vi "Periodic Tasks.vi"(8 "error in (no error)":errorcluster) -> ()   [LabVIEW 2011]
doc: "This VI runs in parallel to other tasks. It can contain as many user-defined periodic loops as you need. These can carry out PID or other sorts of timed response."
uses:
  <vilib>/Rock Robotics/SystemInterfaces/Utilities/FPGA_UtilitiesLED State.ctl
  <vilib>/Rock Robotics/SystemInterfaces/Utilities/FPGA_UtilitiesLED Source.ctl
  Robot Global Data.vi
panel:
  out "Autonomous Switch":dbl
  out "Encoder Direction 4":string="Backward"
  out "Encoder Alarm Status 4":string="Encoder Moving"
  in  "stop 4":bool
  out "Encoder Distance 4":dbl
  out "Encoder Rate (distance/sec) 4":dbl
  out "Encoder Direction 3":string="Backward"
  out "Encoder Alarm Status 3":string="Encoder Moving"
  in  "Reset Encoder? 3":bool
  in  "stop 3":bool
  out "Encoder Distance 3":dbl
  out "Encoder Rate (distance/sec) 3":dbl
  out "Encoder Direction 2":string="Forward"
  out "Encoder Alarm Status 2":string="Encoder Stopped"
  in  "Reset Encoder? 2":bool
  in  "stop 2":bool
  out "Encoder Distance 2":dbl=1.0
  out "Encoder Rate (distance/sec) 2":dbl
  out "Encoder Direction":string="Forward"
  out "Encoder Alarm Status":string="Encoder Stopped"
  in  "Reset Encoder?":bool
  in  "stop":bool
  out "Encoder Distance":dbl=1.0
  out "Encoder Rate (distance/sec)":dbl
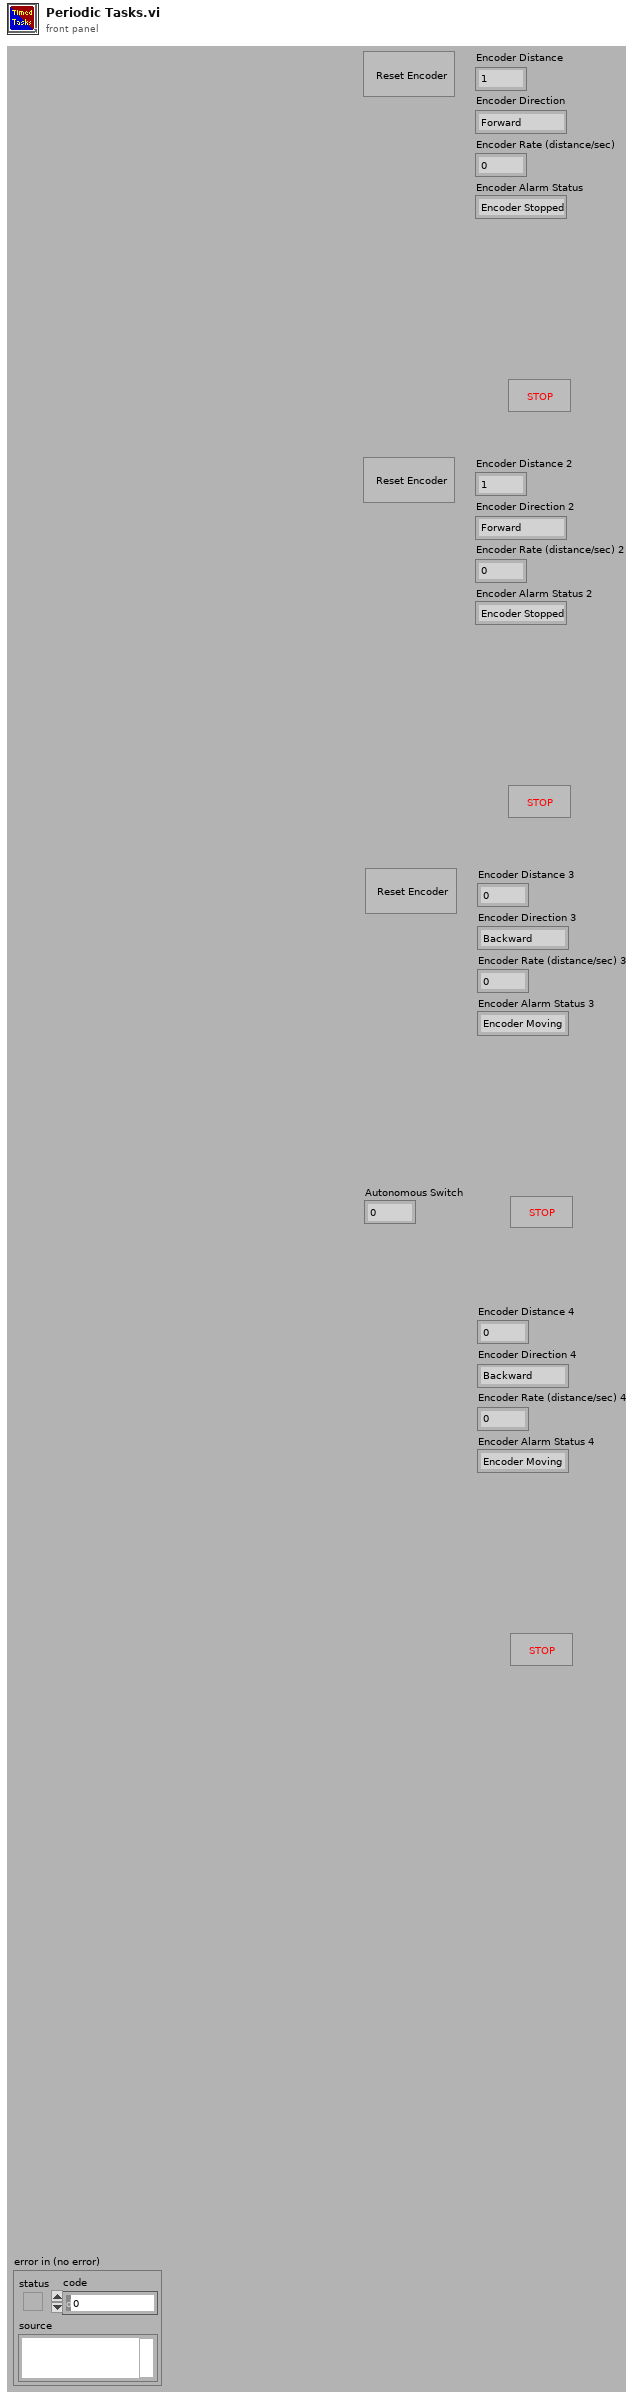
[diagram p1: front panel]
types:
  T1 = typedef "FPGA_UtilitiesLED State.ctl" = enum16{"Off", "On", "Toggle"}
  T2 = typedef "FPGA_UtilitiesLED Source.ctl" = enum16{"User LED", "FPGA LED"}
  T3 = enum16{"Shoot", "Load", "Arm", "Nothing", "Reverse", "ShootAll"}
  T4 = typedef "WPI_DigitalInputDevRef.ctl" = cluster{"DevStatus":errorcluster, "DIO Channel":T5, "Digital Module":T6}
  T5 = typedef "FPGA_DIOChannel.ctl" = enum8{"DIO 1", "DIO 2", "DIO 3", "DIO 4", "DIO 5", "DIO 6", "DIO 7", "DIO 8", "DIO 9", "DIO 10", "DIO 11", "DIO 12", "DIO 13", "DIO 14", "Invalid"}
  T6 = typedef "FPGA_TypedefDigitalModule.ctl" = enum16{"Digital Module 1", "Digital Module 2"}
  T7 = typedef "WPI_EncoderDevRef.ctl" = cluster{"DevStatus":errorcluster, "EncoderIndex":T8, "CounterIndex":T9, "DistancePerCount":dbl, "Decoding Type":T10}
  T8 = typedef "FPGA_EncoderIdx.ctl" = enum8{"Enc 0", "Enc 1", "Enc 2", "Enc 3", "Invalid"}
  T9 = typedef "FPGA_CounterCtrSystemIndex.ctl" = enum8{"Ctr 0", "Ctr 1", "Ctr 2", "Ctr 3", "Ctr 4", "Ctr 5", "Ctr 6", "Ctr 7", "Invalid"}
  T10 = typedef "WPI_EncoderType.ctl" = enum16{"1x", "2x", "4x"}
  T11 = typedef "WPI_MotorControlDeviceRef.ctl" = cluster{"DeviceStatus":errorcluster, "Type":enum16{"PWM", "CAN"}, "PWM":cluster{"Digital Module":T6, "PWM Channel":T12, "DeadBand":T13}, "CAN":cluster{"Device Number":u8, "Control Mode":T14, "Semaphore":T15, "Max Vout":dbl}, "Invert":bool, "TransformRef":T16, "InvTransformRef":T16}
  T12 = typedef "FPGA_DIOPWMChannel.ctl" = enum8{"PWM 1", "PWM 2", "PWM 3", "PWM 4", "PWM 5", "PWM 6", "PWM 7", "PWM 8", "PWM 9", "PWM 10", "Invalid"}
  T13 = typedef "WPI_PWMDeadband.ctl" = cluster{"Name":string, "maxPositivePwm":i32, "minPositivePwm":i32, "centerPwm":i32, "maxNegativePwm":i32, "minNegativePwm":i32, "angularRange":u16}
  T14 = typedef "WPI_CANJaguar_ControlMode.ctl" = enum8{"Percent VBus", "Current", "Speed", "Position", "Voltage"}
  T15 = typedef "Semaphore RefNum" = refnum<k1>
  T16 = typedef "WPI_PWMTransform_ConPane.ctl" = refnum<vi>
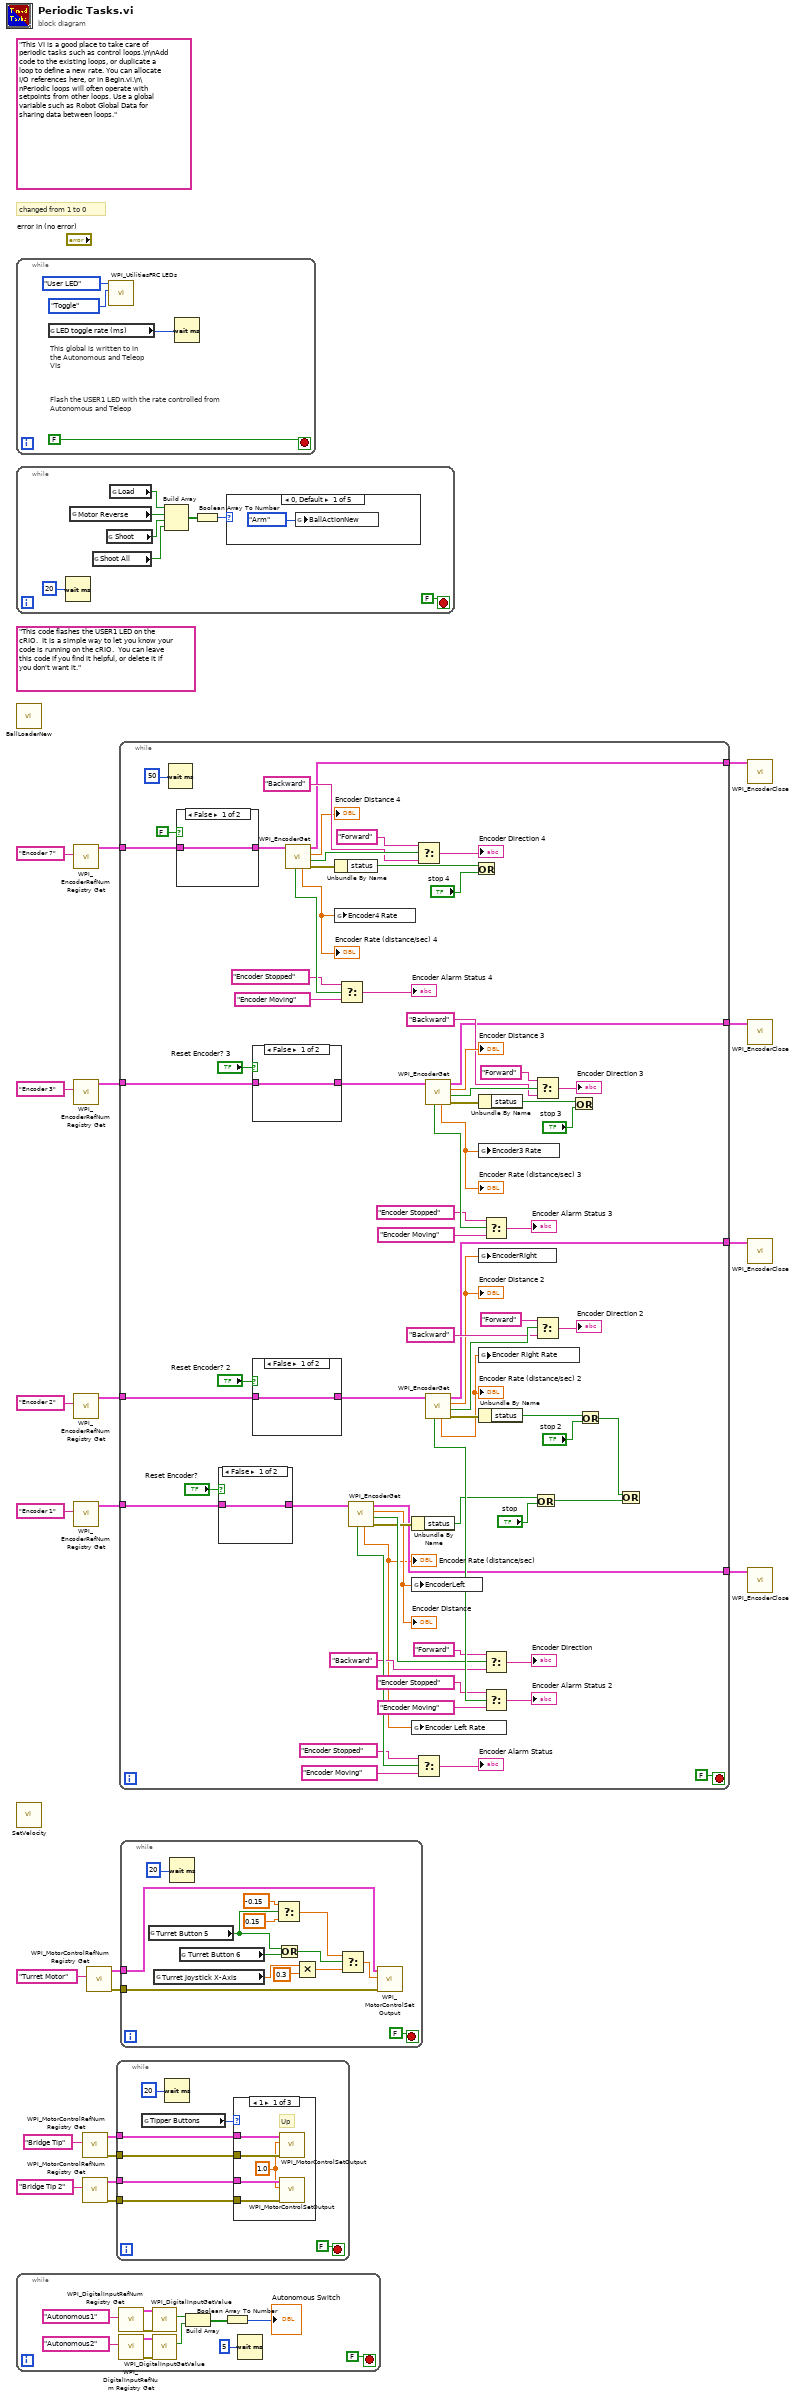
[diagram p0: block diagram]
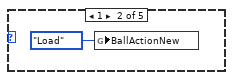
[diagram p2: hidden frame]
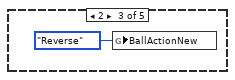
[diagram p3: hidden frame]
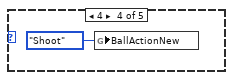
[diagram p4: hidden frame]
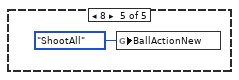
[diagram p5: hidden frame]
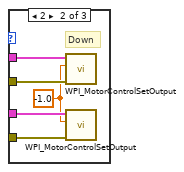
[diagram p6: hidden frame]
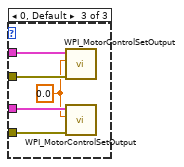
[diagram p7: hidden frame]
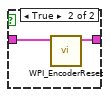
[diagram p8: hidden frame]
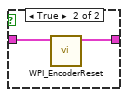
[diagram p9: hidden frame]
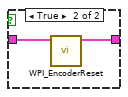
[diagram p10: hidden frame]
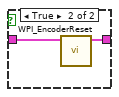
[diagram p11: hidden frame]
diagram:
  (unwired) "This VI is a good place to take care of periodic tasks such as control loops.\n\nAdd code to the existing loops, or duplicate a loop to define a new rate. You can allocate I/O references here, or in Begin.vi.\n\nPeriodic loops will often operate with setpoints from other loops. Use a global variable such as Robot Global Data for sharing data between loops."
  (unwired) "This code flashes the USER1 LED on the cRIO.  It is a simple way to let you know your code is running on the cRIO.  You can leave this code if you find it helpful, or delete it if you don't want it."
  # "changed from 1 to 0"
  n1 = while {
    stop <- FALSE stop-if-true
    # "This global is written to in the Autonomous and Teleop VIs"
    # "Flash the USER1 LED with the rate controlled from Autonomous and Teleop"
    n2 = global read "Robot Global Data.vi" "LED toggle rate (ms)"() -> (w22:u32)
    n3 = call <vilib>:"WPI_UtilitiesFRC LEDs.vi"("State"=FPGA_UtilitiesLED_State."Toggle", "LED Type"=FPGA_UtilitiesLED_Source."User LED") -> ()  [unwired: 1 in, 9 out]
    n4 = Wait (ms)(milliseconds to wait=w22) -> ()  [unwired: 1 out]
  }
  n5 = while {
    stop <- FALSE stop-if-true
    n6 = Wait (ms)(milliseconds to wait=u32 20) -> ()  [unwired: 1 out]
    n7 = global read "Robot Global Data.vi" "Motor Reverse"() -> (w31:bool)
    n8 = global read "Robot Global Data.vi" "Shoot All"() -> (w29:bool)
    n9 = global read "Robot Global Data.vi" "Shoot"() -> (w30:bool)
    n10 = global read "Robot Global Data.vi" "Load"() -> (w32:bool)
    n11 = Build Array(w32, w31, w30, w29) -> (w33:bool[])
    n12 = Boolean Array To Number(Boolean array=w33) -> (number=w28:u32)
    n13 = case shown="0, Default" w28 {
      frame 0, Default {
        n14 = global write "Robot Global Data.vi" "BallActionNew"(T3."Arm" ("BallActionNew")) -> ()
      }
      frame 1 {
        n15 = global write "Robot Global Data.vi" "BallActionNew"(T3."Load" ("BallActionNew")) -> ()
      }
      frame 2 {
        n16 = global write "Robot Global Data.vi" "BallActionNew"(T3."Reverse" ("BallActionNew")) -> ()
      }
      frame 4 {
        n17 = global write "Robot Global Data.vi" "BallActionNew"(T3."Shoot" ("BallActionNew")) -> ()
      }
      frame 8 {
        n18 = global write "Robot Global Data.vi" "BallActionNew"(T3."ShootAll" ("BallActionNew")) -> ()
      }
    }
  }
  n19 = call "BallLoaderNew.vi"() -> ()  [unwired: 12 in]
  n20 = call "SetVelocity.vi"() -> ()  [unwired: 12 in]
  n21 = while {
    stop <- FALSE stop-if-true
    n22 = call <vilib>:"WPI_DigitalInputRefNum Registry Get.vi"("refnum name"="Autonomous1") -> ("error out"=w48:errorcluster, "DigitalInputDevRef"=w47:T4)  [unwired: 9 in]
    n23 = call <vilib>:"WPI_DigitalInputRefNum Registry Get.vi"("refnum name"="Autonomous2") -> ("error out"=w45:errorcluster, "DigitalInputDevRef"=w46:T4)  [unwired: 9 in]
    n24 = call <vilib>:"WPI_DigitalInputGetValue.vi"("error in (no error)"=w48, "DigitalInputDevRef"=w47) -> ("Value"=w49:bool)  [unwired: 7 in, 2 out]
    n25 = call <vilib>:"WPI_DigitalInputGetValue.vi"("error in (no error)"=w45, "DigitalInputDevRef"=w46) -> ("Value"=w50:bool)  [unwired: 7 in, 2 out]
    n26 = Build Array(w49, w50) -> (w42:bool[])
    n27 = Boolean Array To Number(Boolean array=w42) -> (number=→"Autonomous Switch":u32)
    n28 = Wait (ms)(milliseconds to wait=u32 5) -> ()  [unwired: 1 out]
  }
  n29 = call <vilib>:"WPI_EncoderRefNum Registry Get.vi"("refnum name"="Encoder 7") -> ("EncoderDevRef"=w20:T7)  [unwired: 9 in, 1 out]
  n30 = call <vilib>:"WPI_EncoderRefNum Registry Get.vi"("refnum name"="Encoder 3") -> ("EncoderDevRef"=w17:T7)  [unwired: 9 in, 1 out]
  n31 = call <vilib>:"WPI_EncoderRefNum Registry Get.vi"("refnum name"="Encoder 2") -> ("EncoderDevRef"=w13:T7)  [unwired: 9 in, 1 out]
  n32 = call <vilib>:"WPI_EncoderRefNum Registry Get.vi"("refnum name"="Encoder 1") -> ("EncoderDevRef"=w11:T7)  [unwired: 9 in, 1 out]
  n33 = call <vilib>:"WPI_MotorControlRefNum Registry Get.vi"("refnum name"="Bridge Tip") -> ("error out"=w4:errorcluster, "MotorControlDevRef"=w5:T11)  [unwired: 9 in]
  n34 = call <vilib>:"WPI_MotorControlRefNum Registry Get.vi"("refnum name"="Bridge Tip 2") -> ("error out"=w1:errorcluster, "MotorControlDevRef"=w2:T11)  [unwired: 9 in]
  n35 = call <vilib>:"WPI_MotorControlRefNum Registry Get.vi"("refnum name"="Turret Motor") -> ("error out"=w7:errorcluster, "MotorControlDevRef"=w8:T11)  [unwired: 9 in]
  n36 = while {
    tunnel: w5 -> [w54]
    tunnel: w4 -> [w53]
    tunnel: w2 -> [w52]
    tunnel: w1 -> [w51]
    stop <- FALSE stop-if-true
    n37 = global read "Robot Global Data.vi" "Tipper Buttons"() -> (w57:i32)
    n38 = Wait (ms)(milliseconds to wait=u32 20) -> ()  [unwired: 1 out]
    n39 = case shown="1" w57 {
      tunnel: w54 -> [w62 w67 w72]
      tunnel: w53 -> [w61 w66 w71]
      tunnel: w52 -> [w59 w65 w70]
      tunnel: w51 -> [w60 w64 w69]
      frame 1 {
        w58 = 1.0 ("Output")
        # "Up"
        n40 = call <vilib>:"WPI_MotorControlSetOutput.vi"("error in (no error)"=w61, "Output"=w58, "MotorControlDevRef"=w62) -> ()  [unwired: 7 in, 2 out]
        n41 = call <vilib>:"WPI_MotorControlSetOutput.vi"("error in (no error)"=w60, "Output"=w58, "MotorControlDevRef"=w59) -> ()  [unwired: 7 in, 2 out]
      }
      frame 2 {
        w63 = -1.0 ("Output")
        # "Down"
        n42 = call <vilib>:"WPI_MotorControlSetOutput.vi"("error in (no error)"=w66, "Output"=w63, "MotorControlDevRef"=w67) -> ()  [unwired: 7 in, 2 out]
        n43 = call <vilib>:"WPI_MotorControlSetOutput.vi"("error in (no error)"=w64, "Output"=w63, "MotorControlDevRef"=w65) -> ()  [unwired: 7 in, 2 out]
      }
      frame 0, Default {
        w68 = 0.0 ("Output")
        n44 = call <vilib>:"WPI_MotorControlSetOutput.vi"("error in (no error)"=w71, "Output"=w68, "MotorControlDevRef"=w72) -> ()  [unwired: 7 in, 2 out]
        n45 = call <vilib>:"WPI_MotorControlSetOutput.vi"("error in (no error)"=w69, "Output"=w68, "MotorControlDevRef"=w70) -> ()  [unwired: 7 in, 2 out]
      }
    }
  }
  n46 = while {
    tunnel: w20 -> [w88]
    tunnel: [w87] -> w19
    tunnel: w17 -> [w86]
    tunnel: [w85] -> w16
    tunnel: [w84] -> w15
    tunnel: w13 -> [w83]
    tunnel: w11 -> [w82]
    tunnel: [w81] -> w10
    stop <- FALSE stop-if-true
    n47 = Wait (ms)(milliseconds to wait=u32 50) -> ()  [unwired: 1 out]
    n48 = case shown="False" FALSE {
      tunnel: w88 -> [w154 w156]
      tunnel: [w154 w155] -> w142
      frame False {
      }
      frame True {
        n49 = call <vilib>:"WPI_EncoderReset.vi"("EncoderDevRef"=w156) -> ("EncoderDevRef"=w155:T7)  [unwired: 1 in, 9 out]
      }
    }
    n50 = case shown="False" "Reset Encoder?" {
      tunnel: w82 -> [w145 w147]
      tunnel: [w145 w146] -> w101
      frame False {
      }
      frame True {
        n51 = call <vilib>:"WPI_EncoderReset.vi"("EncoderDevRef"=w147) -> ("EncoderDevRef"=w146:T7)  [unwired: 1 in, 9 out]
      }
    }
    n52 = case shown="False" "Reset Encoder? 3" {
      tunnel: w86 -> [w151 w153]
      tunnel: [w151 w152] -> w129
      frame False {
      }
      frame True {
        n53 = call <vilib>:"WPI_EncoderReset.vi"("EncoderDevRef"=w153) -> ("EncoderDevRef"=w152:T7)  [unwired: 1 in, 9 out]
      }
    }
    n54 = case shown="False" "Reset Encoder? 2" {
      tunnel: w83 -> [w148 w150]
      tunnel: [w148 w149] -> w115
      frame False {
      }
      frame True {
        n55 = call <vilib>:"WPI_EncoderReset.vi"("EncoderDevRef"=w150) -> ("EncoderDevRef"=w149:T7)  [unwired: 1 in, 9 out]
      }
    }
    n56 = call <vilib>:"WPI_EncoderGet.vi"("EncoderDevRef"=w142) -> ("error out"=w139:errorcluster, "Direction"=w141:bool, "Distance"=→"Encoder Distance 4":dbl, "EncoderDevRef"=w87:T7, "Rate"=w132:dbl, "Stopped"=w140:bool)  [unwired: 1 in, 4 out]
    "Encoder Rate (distance/sec) 4" <- w132
    n57 = Unbundle By Name(w139) -> ("status"=w137:bool)
    n58 = global write "Robot Global Data.vi" "Encoder4 Rate"(w132) -> ()
    n59 = Select(t="Encoder Stopped", s=w140, f="Encoder Moving") -> (s? t:f=→"Encoder Alarm Status 4":string)
    n60 = call <vilib>:"WPI_EncoderGet.vi"("EncoderDevRef"=w101) -> ("error out"=w97:errorcluster, "Direction"=w100:bool, "Distance"=w77:dbl, "EncoderDevRef"=w81:T7, "Rate"=w74:dbl, "Stopped"=w99:bool)  [unwired: 1 in, 4 out]
    "Encoder Distance" <- w77
    "Encoder Rate (distance/sec)" <- w74
    n61 = Unbundle By Name(w97) -> ("status"=w95:bool)
    n62 = global write "Robot Global Data.vi" "EncoderLeft"(w77) -> ()
    n63 = global write "Robot Global Data.vi" "Encoder Left Rate"(w74) -> ()
    n64 = Select(t="Forward", s=w141, f="Backward") -> (s? t:f=→"Encoder Direction 4":string)
    n65 = Select(t="Encoder Stopped", s=w99, f="Encoder Moving") -> (s? t:f=→"Encoder Alarm Status":string)
    n66 = call <vilib>:"WPI_EncoderGet.vi"("EncoderDevRef"=w129) -> ("error out"=w124:errorcluster, "Direction"=w128:bool, "Distance"=→"Encoder Distance 3":dbl, "EncoderDevRef"=w85:T7, "Rate"=w75:dbl, "Stopped"=w127:bool)  [unwired: 1 in, 4 out]
    "Encoder Rate (distance/sec) 3" <- w75
    n67 = call <vilib>:"WPI_EncoderGet.vi"("EncoderDevRef"=w115) -> ("error out"=w111:errorcluster, "Direction"=w114:bool, "Distance"=w76:dbl, "EncoderDevRef"=w84:T7, "Rate"=w73:dbl, "Stopped"=w113:bool)  [unwired: 1 in, 4 out]
    "Encoder Distance 2" <- w76
    "Encoder Rate (distance/sec) 2" <- w73
    n68 = Or(x=w137, y="stop 4") -> ()  [unwired: 1 out]
    n69 = Unbundle By Name(w124) -> ("status"=w122:bool)
    n70 = global write "Robot Global Data.vi" "Encoder3 Rate"(w75) -> ()
    n71 = global write "Robot Global Data.vi" "EncoderRight"(w76) -> ()
    n72 = global write "Robot Global Data.vi" "Encoder Right Rate"(w73) -> ()
    n73 = Unbundle By Name(w111) -> ("status"=w109:bool)
    n74 = Select(t="Encoder Stopped", s=w127, f="Encoder Moving") -> (s? t:f=→"Encoder Alarm Status 3":string)
    n75 = Select(t="Forward", s=w100, f="Backward") -> (s? t:f=→"Encoder Direction":string)
    n76 = Select(t="Encoder Stopped", s=w113, f="Encoder Moving") -> (s? t:f=→"Encoder Alarm Status 2":string)
    n77 = Or(x=w95, y="stop") -> (x .or. y?=w89:bool)
    n78 = Select(t="Forward", s=w128, f="Backward") -> (s? t:f=→"Encoder Direction 3":string)
    n79 = Select(t="Forward", s=w114, f="Backward") -> (s? t:f=→"Encoder Direction 2":string)
    n80 = Or(x=w122, y="stop 3") -> ()  [unwired: 1 out]
    n81 = Or(x=w109, y="stop 2") -> (x .or. y?=w90:bool)
    n82 = Or(x=w90, y=w89) -> ()  [unwired: 1 out]
  }
  n83 = while {
    tunnel: w8 -> [w167]
    tunnel: w7 -> [w166]
    stop <- FALSE stop-if-true
    n84 = global read "Robot Global Data.vi" "Turret Button 5"() -> (w160:bool)
    n85 = global read "Robot Global Data.vi" "Turret Joystick X-Axis"() -> (w170:dbl)
    n86 = Wait (ms)(milliseconds to wait=u32 20) -> ()  [unwired: 1 out]
    n87 = global read "Robot Global Data.vi" "Turret Button 6"() -> (w162:bool)
    n88 = Select(t=-0.15, s=w160, f=0.15) -> (s? t:f=w157:dbl)
    n89 = Or(x=w160, y=w162) -> (x .or. y?=w161:bool)
    n90 = Multiply(x=w170, y=0.3) -> (x*y=w163:dbl)
    n91 = Select(t=w157, s=w161, f=w163) -> (s? t:f=w164:dbl)
    n92 = call <vilib>:"WPI_MotorControlSetOutput.vi"("error in (no error)"=w166, "Output"=w164, "MotorControlDevRef"=w167) -> ()  [unwired: 7 in, 2 out]
  }
  n93 = call <vilib>:"WPI_EncoderClose.vi"("EncoderDevRef"=w19) -> ()  [unwired: 2 in, 9 out]
  n94 = call <vilib>:"WPI_EncoderClose.vi"("EncoderDevRef"=w16) -> ()  [unwired: 2 in, 9 out]
  n95 = call <vilib>:"WPI_EncoderClose.vi"("EncoderDevRef"=w15) -> ()  [unwired: 2 in, 9 out]
  n96 = call <vilib>:"WPI_EncoderClose.vi"("EncoderDevRef"=w10) -> ()  [unwired: 2 in, 9 out]
